vi "Manual.vi"(8 "error in (no error)":errorcluster, 10 "shutdown":refnum<user-event>, 11 "String":string) -> (0 "error out":errorcluster)   [LabVIEW 2025]
uses:
  Classes/Dynamic-System/dynamic system selection.ctl
  Classes/Dynamic-System/controller selection.ctl
  Classes/Dynamic-System/Dynamic-System.lvclass
  Classes/mass-spring-damper/mass-spring-damper.lvclass
  C:/Users/grove/Desktop/LabVIEW/Git/dynamic-systems/Classes/Dynamic-System/Dynamic-System.lvclass
  Classes/water-tank/water-tank.lvclass
  <vilib>/Handler Framework/CmdQueue/Enqueue Single.vi
  <vilib>/Handler Framework/Handler Framework.lvlib
  C:/Users/grove/Desktop/LabVIEW/Git/dynamic-systems/Classes/mass-spring-damper/mass-spring-damper.lvclass
  C:/Users/grove/Desktop/LabVIEW/Git/dynamic-systems/Classes/water-tank/water-tank.lvclass
panel:
  in  "PID gains":T1
  in  "Update PID":bool
  in  "Dynamic System":T2
  in  "Controller Selection":T3=enum."PID"
  out "XY Plot":cluster{"Time":dbl[], "Reference":dbl[]}[](graph)
  in  "Run Sim":bool
  # "MANUAL"
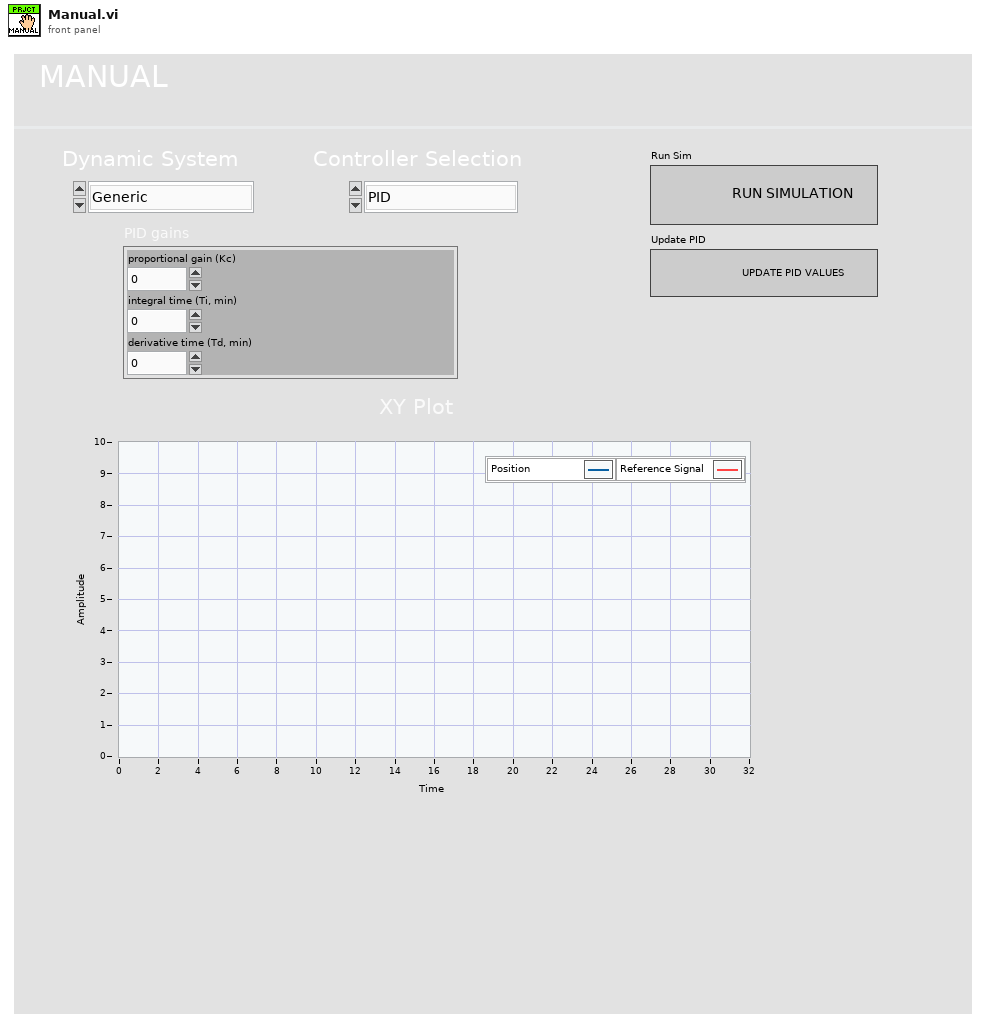
[diagram p1: front panel]
types:
  T1 = cluster{"proportional gain (Kc)":dbl, "integral time (Ti, min)":dbl, "derivative time (Td, min)":dbl}
  T2 = typedef "dynamic system selection.ctl" = enum16{"Generic", "Mass Spring Damper", "Water Tank", "RLC Circuit"}
  T3 = typedef "controller selection.ctl" = enum16{"No Control", "PID", "On Off"}
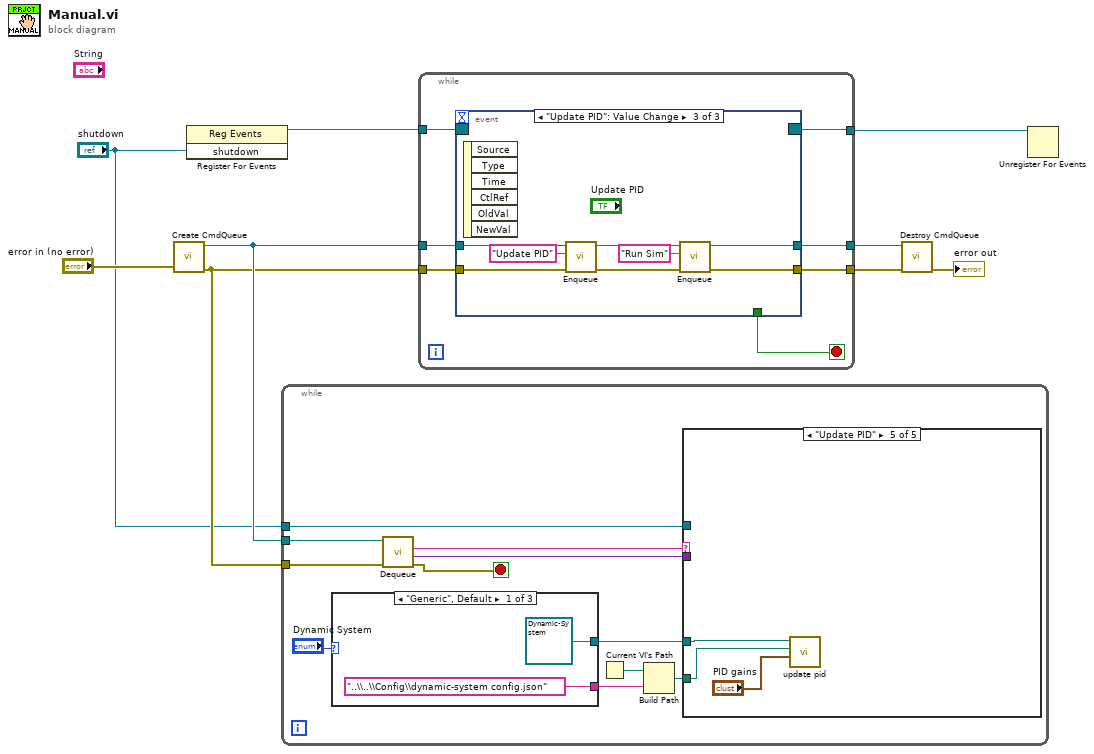
[diagram p0: block diagram]
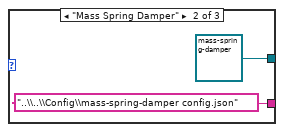
[diagram p2: hidden frame]
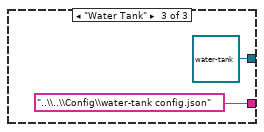
[diagram p3: hidden frame]
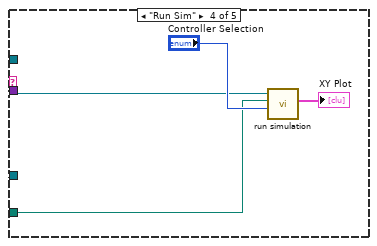
[diagram p7: hidden frame]
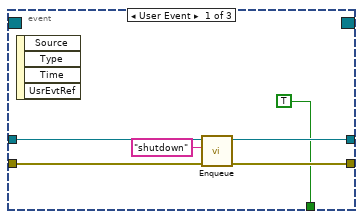
[diagram p8: hidden frame]
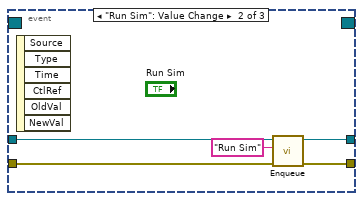
[diagram p9: hidden frame]
diagram:
  n1 = call <vilib>:"Create CmdQueue.vi"("error in (no error)"="error in (no error)") -> ("error out"=w6:errorcluster, "CmdQueue out"=w7:refnum<queue>)  [unwired: 9 in]
  n2 = register-events("shutdown") -> (reference out=w5:refnum<event-registration>)  [unwired: 2 in, 1 out]
  n3 = while {
    tunnel: w7 -> [w20]
    tunnel: w6 -> [w16]
    tunnel: "shutdown" -> [w15]
    stop <- w17 stop-if-true
    n4 = case shown="\"Generic\", Default" "Dynamic System" {
      tunnel: [refnum<class "Dynamic-System.lvclass"> refnum ("Dynamic-System.lvclass") refnum<class "mass-spring-damper.lvclass"> refnum ("mass-spring-damper.lvclass") refnum<class "water-tank.lvclass"> refnum ("water-tank.lvclass")] -> w13
      tunnel: ["..\\..\\Config\\dynamic-system config.json" "..\\..\\Config\\mass-spring-damper config.json" "..\\..\\Config\\water-tank config.json"] -> w11
      frame "Generic", Default {
      }
      frame "Mass Spring Damper" {
      }
      frame "Water Tank" {
      }
    }
    n5 = call <vilib>:"Dequeue.vi"("error in (no error)"=w16, "CmdQueue in"=w20) -> ("error out"=w17:errorcluster, "value"=w18:variant, "cmd"=w19:string)  [unwired: 5 in, 2 out]
    n6 = Current VI's Path() -> (path=w12:path)
    n7 = Build Path(base path=w12, name or relative path=w11) -> (appended path=w10:path)
    n8 = case shown="\"Update PID\"" w19 {
      tunnel: w18 -> [_ _ _ _ _]
      tunnel: w15 -> [_ _ _ _ _]
      tunnel: w13 -> [_ _ _ w28 w33]
      tunnel: w10 -> [_ _ _ w27 w32]
      frame "False", Default {
      }
      frame "init" {
      }
      frame "shutdown" {
      }
      frame "Run Sim" {
        n9 = call-dynamic "run simulation.vi"("Controller Selection"="Controller Selection", "Config Path"=w27, "Dynamic-System in"=w28) -> ("XY Plot"=→"XY Plot":cluster{"Time":dbl[], "Reference":dbl[]}[])  [unwired: 6 in, 2 out]
      }
      frame "Update PID" {
        n10 = call-dynamic "update pid.vi"("PID gains"="PID gains", "config path"=w32, "Dynamic-System in"=w33) -> ()  [unwired: 7 in, 2 out]
      }
    }
  }
  n11 = while {
    tunnel: w7 -> [w40]
    tunnel: [w39] -> w9
    tunnel: w6 -> [w38]
    tunnel: [w37] -> w8
    tunnel: w5 -> [w35]
    tunnel: [w34] -> w4
    stop <- w36 stop-if-true
    n12 = event shown="[2] \"Update PID\": Value Change" {
      selector: w35 -> [_ _ _]
      dyn-events: [_ _ _] -> w34
      timeout: _ -> [_ _ _]
      tunnel: w40 -> [w46 w49 w59]
      tunnel: [w45 w51 w53] -> w39
      tunnel: w38 -> [w44 w48 w58]
      tunnel: [w43 w50 w52] -> w37
      tunnel: [TRUE ("Discard?") _ _] -> w36
      event User Event {
        n13 = event-data() -> ()  [unwired: 1 in, 4 out]
        n14 = call-poly <vilib>:"Enqueue.vi"("error in (no error)"=w44, "Command"="shutdown", "CmdQueue in"=w46) -> ("error out"=w43:errorcluster, "CmdQueue out"=w45:refnum<queue>)  [unwired: 7 in]
      }
      event "Run Sim": Value Change {
        n15 = event-data() -> ()  [unwired: 1 in, 6 out]
        n16 = call-poly <vilib>:"Enqueue.vi"("error in (no error)"=w48, "Command"="Run Sim", "CmdQueue in"=w49) -> ("error out"=w50:errorcluster, "CmdQueue out"=w51:refnum<queue>)  [unwired: 7 in]
      }
      event "Update PID": Value Change {
        n17 = event-data() -> ()  [unwired: 1 in, 6 out]
        n18 = call-poly <vilib>:"Enqueue.vi"("error in (no error)"=w58, "Command"="Update PID", "CmdQueue in"=w59) -> ("error out"=w55:errorcluster, "CmdQueue out"=w56:refnum<queue>)  [unwired: 7 in]
        n19 = call-poly <vilib>:"Enqueue.vi"("error in (no error)"=w55, "Command"="Run Sim", "CmdQueue in"=w56) -> ("error out"=w52:errorcluster, "CmdQueue out"=w53:refnum<queue>)  [unwired: 7 in]
      }
    }
  }
  n20 = call <vilib>:"Destroy CmdQueue.vi"("error in (no error)"=w8, "CmdQueue in"=w9) -> ("error out"=→"error out":errorcluster)  [unwired: 9 in]
  n21 = Unregister For Events(event registration refnum=w4) -> ()  [unwired: 1 in, 1 out]
